vi "get_power_reading.vi"(0 "reference in":refnum<k7>, 5 "hDevice":i32, 9 "channel":i32, 11 "error in (no error)":errorcluster) -> (4 "reference out":refnum<k7>, 6 "hDevice out":i32, 10 "channel out":i32, 12 "Power / J":dbl, 13 "Timestamp":dbl, 14 "Status":i32, 15 "error out":errorcluster)   [LabVIEW 2020]
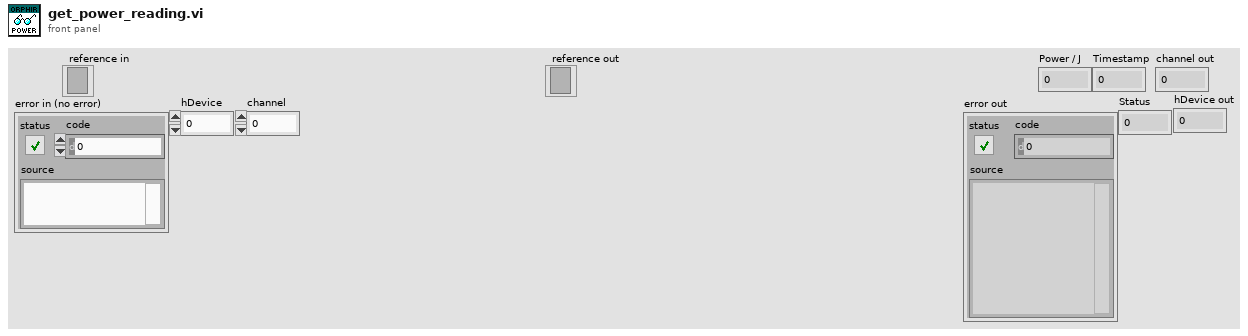
[diagram p1: front panel]
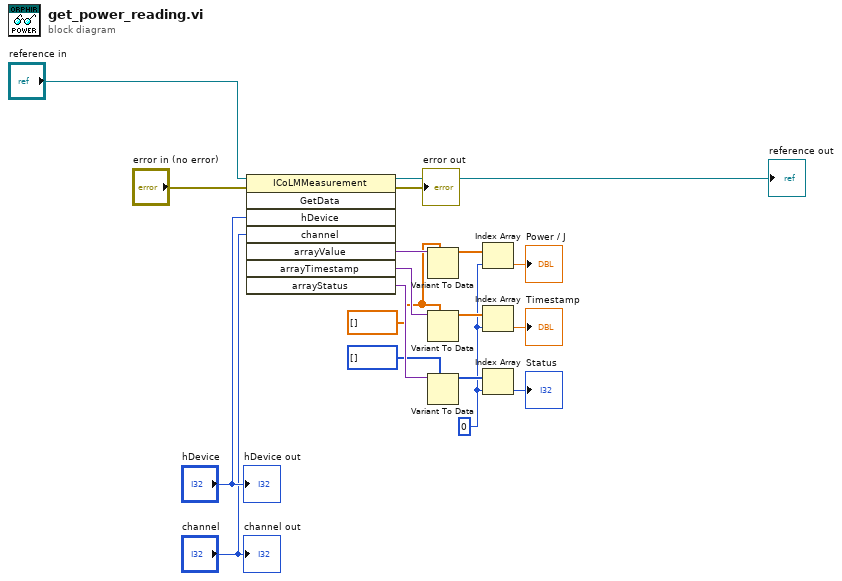
[diagram p0: block diagram]
diagram:
  w6 = 0 ("index")
  w10 = dbl[] []
  n1 = invoke class="ICoLMMeasurement" method="GetData"(reference="reference in", error in="error in (no error)", "hDevice"="hDevice", "channel"="channel") -> (reference out=→"reference out":refnum<k7>, error out=→"error out":errorcluster, "arrayValue"=w18:variant, "arrayTimestamp"=w17:variant, "arrayStatus"=w16:variant)  [unwired: 4 in, 3 out]
  n2 = Variant To Data(type=w10, Variant=w18) -> (data=w9:dbl[])  [unwired: 1 in, 1 out]
  n3 = Variant To Data(type=w10, Variant=w17) -> (data=w8:dbl[])  [unwired: 1 in, 1 out]
  n4 = Variant To Data(type=i32[] [], Variant=w16) -> (data=w7:i32[])  [unwired: 1 in, 1 out]
  n5 = Index Array(array=w9, index=w6) -> (element=→"Power / J":dbl)
  n6 = Index Array(array=w8, index=w6) -> (element=→"Timestamp":dbl)
  n7 = Index Array(array=w7, index=w6) -> (element=→"Status":i32)
  "channel out" <- "channel"
  "hDevice out" <- "hDevice"
